vi "circular_feeder.vi"(0 "Shoot":bool, 1 "Limit Switch":bool, 2 "Dt":u32=1000, 3 "Spinning Speed":dbl=3.0) -> (5 "Ready":bool, 6 "Motor Voltage":dbl)   [LabVIEW 2012]
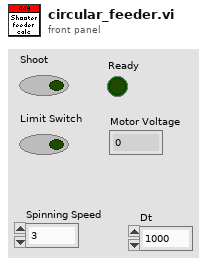
[diagram p1: front panel]
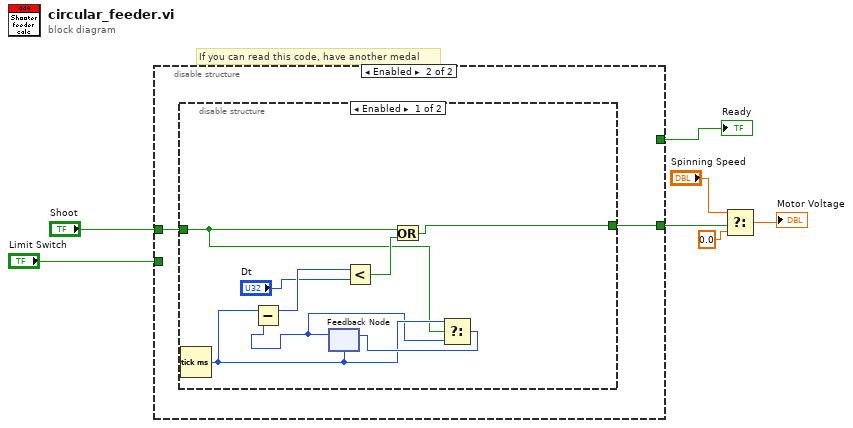
[diagram p0: block diagram]
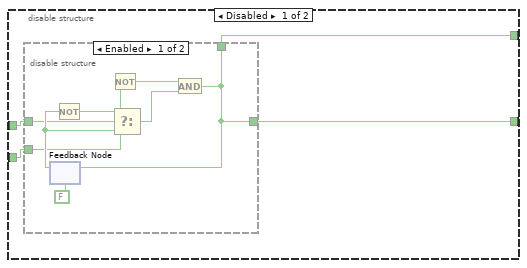
[diagram p2: hidden frame]
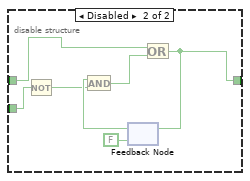
[diagram p3: hidden frame]
diagram:
  # "If you can read this code, have another medal"
  n1 = disable-structure shown="Enabled" {
    disable-tunnel: "Shoot" -> [w11 w27]
    disable-tunnel: "Limit Switch" -> [w10 _]
    disable-tunnel: [w9 _] -> w3
    disable-tunnel: [w8 w28] -> w2
    frame Disabled {
      n2 = disable-structure shown="Enabled" {
        disable-tunnel: w11 -> [w16 w22]
        disable-tunnel: w10 -> [w13 w23]
        disable-tunnel: [w14 _] -> w9
        disable-tunnel: [w14 w25] -> w8
        frame Enabled {
          n3 = feedback #1(FALSE) -> (w18:bool)
          n4 = Not(x=w18) -> (.not. x?=w19:bool)
          n5 = Not(x=w13) -> (.not. x?=w12:bool)
          n6 = Select(t=w19, s=w16, f=w18) -> (s? t:f=w15:bool)
          n7 = And(x=w12, y=w15) -> (x .and. y?=w14:bool)
          n8 = feedback-in #1(w14) -> ()
        }
        frame Disabled {
          n9 = Not(x=w23) -> (.not. x?=w21:bool)
          n10 = feedback #2(FALSE) -> (w24:bool)
          n11 = And(x=w24, y=w21) -> (x .and. y?=w26:bool)
          n12 = Or(x=w22, y=w26) -> (x .or. y?=w25:bool)
          n13 = feedback-in #2(w25) -> ()
        }
      }
    }
    frame Enabled {
      n14 = disable-structure shown="Enabled" {
        disable-tunnel: [w35 w37] -> w28
        disable-tunnel: w27 -> [w29 w37]
        frame Enabled {
          n15 = Tick Count (ms)() -> (millisecond timer value=w33:u32)
          n16 = feedback #3(w33) -> (w32:u32)
          n17 = Subtract(x=w33, y=w32) -> (x-y=w36:u32)
          n18 = Less?(x=w36, y="Dt") -> (x < y?=w30:bool)
          n19 = Or(x=w29, y=w30) -> (x .or. y?=w35:bool)
          n20 = Select(t=w33, s=w29, f=w32) -> (s? t:f=w34:u32)
          n21 = feedback-in #3(w34) -> ()
        }
        frame Disabled {
        }
      }
    }
  }
  "Ready" <- w3
  n22 = Select(t="Spinning Speed", s=w2, f=0.0) -> (s? t:f=→"Motor Voltage":dbl)
